vi "Module - RH_BUJAH.vi"() -> ()   [LabVIEW 2019]
uses:
  Control/State - eFGV.ctl
panel:
  out "Site Name":string="RH BUJAH (34.58 kWp)"
  out "STP-04-STATUS":bool
  out "STP-04-B-IDC":dbl caption="B.Idc" format="%.0f A"
  out "STP-04-B-VDC":dbl caption="B.Vdc" format="%.0f V"
  out "STP-04-A-IDC":dbl caption="A.Idc" format="%.0f A"
  out "STP-04-A-VDC":dbl caption="A.Vdc" format="%.0f V"
  out "STP-04-PAC":dbl caption="Pac" format="%#_g W"
  out "BANK-04-TEMP":dbl caption="T_bat" format="%#_g °C"
  out "BANK-04-IDC":dbl caption="I_bat" format="%#_g A"
  out "BANK-04-VDC":dbl caption="V_bat" format="%#_g V"
  out "BANK-04-SOC":dbl caption="SOC" format="%#_g %"
  out "BANK-03-TEMP":dbl caption="T_bat" format="%#_g °C"
  out "BANK-03-IDC":dbl caption="I_bat" format="%#_g A"
  out "BANK-03-VDC":dbl caption="V_bat" format="%#_g V"
  out "BANK-03-SOC":dbl caption="SOC" format="%#_g %"
  out "SI-M-02-STATUS":bool
  out "SI-M-02-FREQ":dbl caption="FREQ" format="%.0f Hz"
  out "SI-M-02-L3":dbl caption="L3" format="%.0f V"
  out "SI-M-02-L2":dbl caption="L2" format="%.0f V"
  out "SI-M-02-L1":dbl caption="L1" format="%.0f V"
  out "SI-M-02-PAC":dbl caption="Pac" format="%.0f W"
  out "STP-03-STATUS":bool
  out "STP-03-B-IDC":dbl caption="B.Idc" format="%.0f A"
  out "STP-03-B-VDC":dbl caption="B.Vdc" format="%.0f V"
  out "STP-03-A-IDC":dbl caption="A.Idc" format="%.0f A"
  out "STP-03-A-VDC":dbl caption="A.Vdc" format="%.0f V"
  out "STP-03-PAC":dbl caption="Pac" format="%#_g W"
  out "PM-01-STATUS":bool
  out "SI-M-01-STATUS":bool
  out "STP-02-STATUS":bool
  out "STP-01-STATUS":bool
  out "BANK-02-TEMP":dbl caption="T_bat" format="%#_g °C"
  out "BANK-02-IDC":dbl caption="I_bat" format="%#_g A"
  out "BANK-02-VDC":dbl caption="V_bat" format="%#_g V"
  out "BANK-02-SOC":dbl caption="SOC" format="%#_g %"
  out "STP-02-B-IDC":dbl caption="B.Idc" format="%.0f A"
  out "STP-02-B-VDC":dbl caption="B.Vdc" format="%.0f V"
  out "STP-02-A-IDC":dbl caption="A.Idc" format="%.0f A"
  out "STP-02-A-VDC":dbl caption="A.Vdc" format="%.0f V"
  out "STP-02-PAC":dbl caption="Pac" format="%#_g W"
  out "PM-01-FREQ":dbl caption="Freq" format="%.0f Hz"
  out "PM-01-IAC":dbl caption="Iac" format="%.0f A"
  out "PM-01-VAC":dbl caption="Vac" format="%.0f V"
  out "PM-01-PAC":dbl caption="Pac" format="%.0f W"
  out "SI-M-01-FREQ":dbl caption="FREQ" format="%.0f Hz"
  out "SI-M-01-L3":dbl caption="L3" format="%.0f V"
  out "SI-M-01-L2":dbl caption="L2" format="%.0f V"
  out "SI-M-01-L1":dbl caption="L1" format="%.0f V"
  out "SI-M-01-PAC":dbl caption="Pac" format="%.0f W"
  out "BANK-01-TEMP":dbl caption="T_bat" format="%#_g °C"
  out "BANK-01-IDC":dbl caption="I_bat" format="%#_g A"
  out "BANK-01-VDC":dbl caption="V_bat" format="%#_g V"
  out "BANK-01-SOC":dbl caption="SOC" format="%#_g %"
  out "STP-01-B-IDC":dbl caption="B.Idc" format="%.0f A"
  out "STP-01-B-VDC":dbl caption="B.Vdc" format="%.0f V"
  out "STP-01-A-IDC":dbl caption="A.Idc" format="%.0f A"
  out "STP-01-A-VDC":dbl caption="A.Vdc" format="%.0f V"
  out "STP-01-PAC":dbl caption="Pac" format="%.0f W"
  # "BANK-1"
  # "BANK-2"
  # "STP2"
  # "BANK-1"
  # "BANK-2"
  # "STP1"
  # "SI-M"
  # "SI-M"
  # "STP3"
  # "STP4"
  # "PM-01"
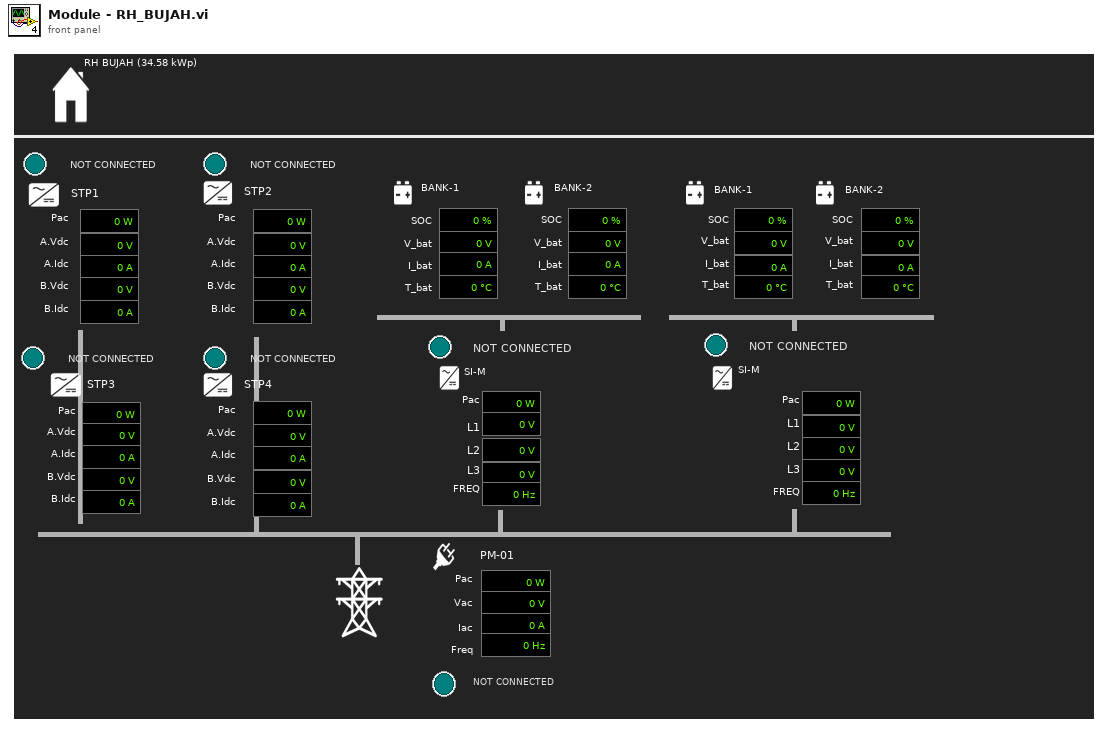
[diagram p1: front panel]
types:
  T1 = typedef "State - eFGV.ctl" = enum16{"Init", "Read", "Write", "Close"}
  T2 = typedef "Device Name.ctl" = enum16{"SB-01", "SB-02", "SB-03", "SB-04", "STP-01", "STP-02", "STP-03", "STP-04", "BANK-01", "BANK-02", "BANK-03", "BANK-04", "SI-M-01", "SI-M-02", "SI-M-03", "SI-M-04", "PM-01", "PM-02", "PM-03", "PM-04"}
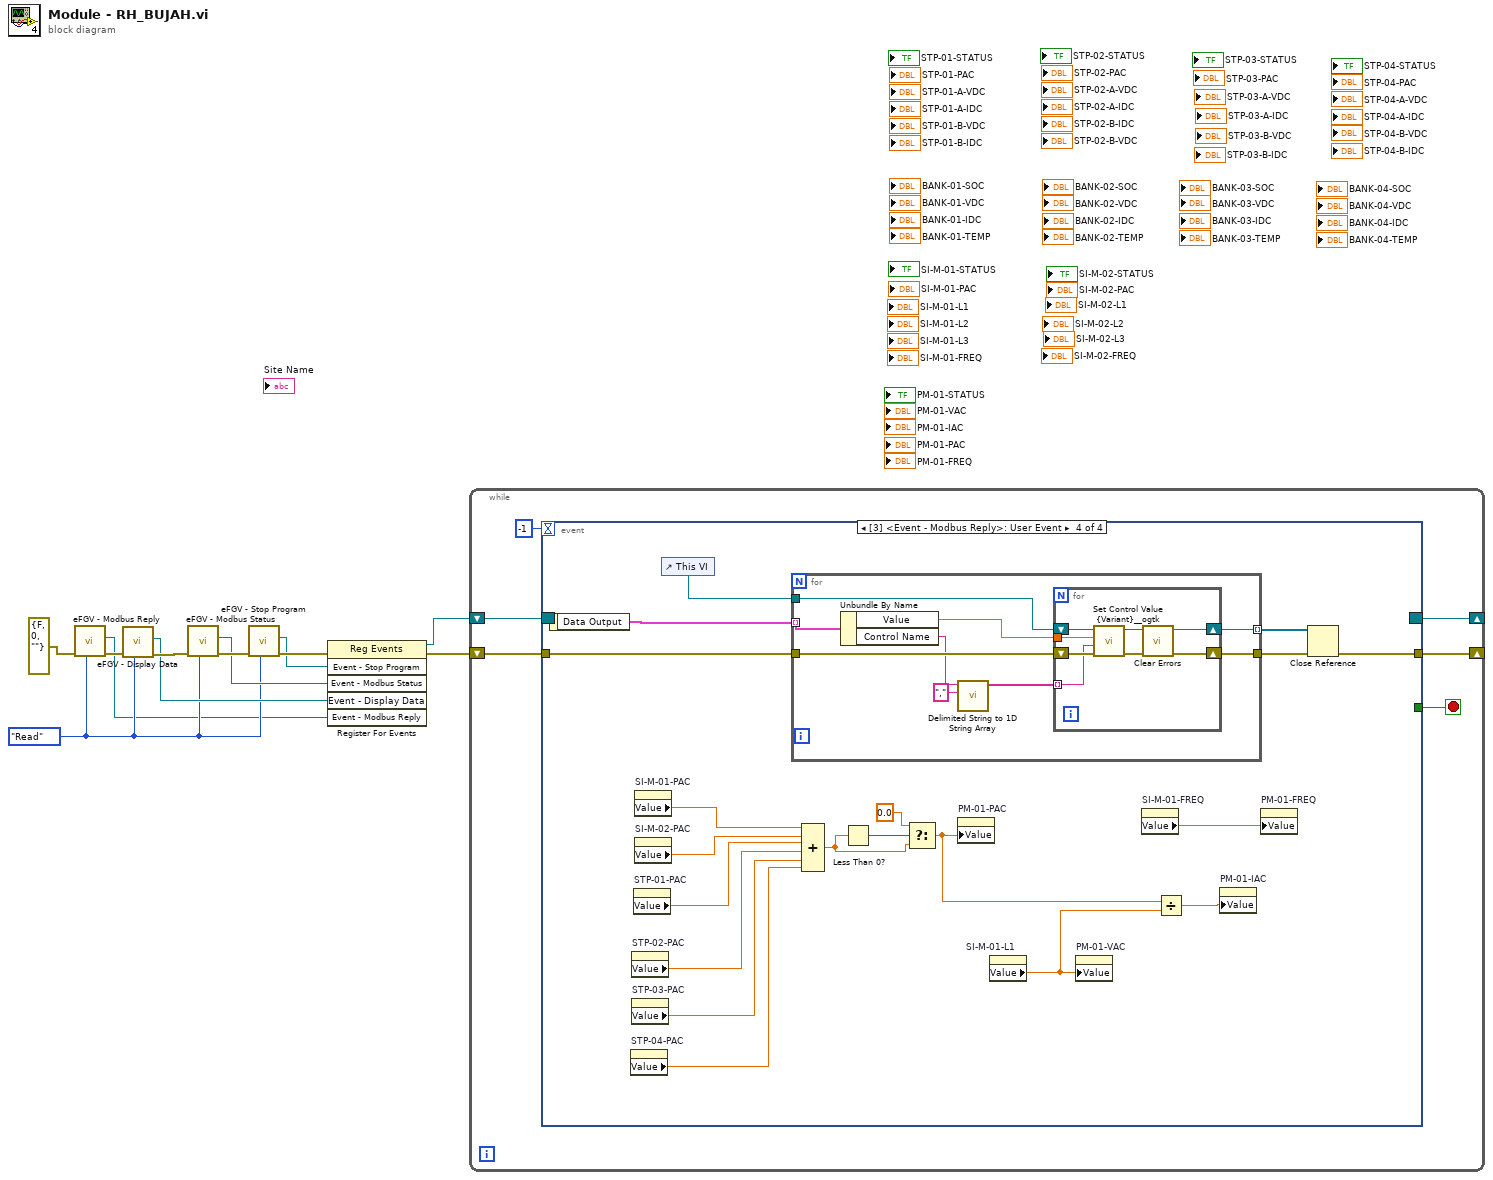
[diagram p0: block diagram]
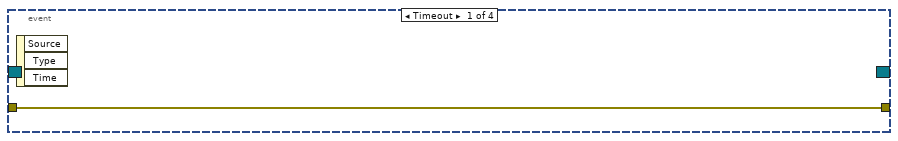
[diagram p2: hidden frame]
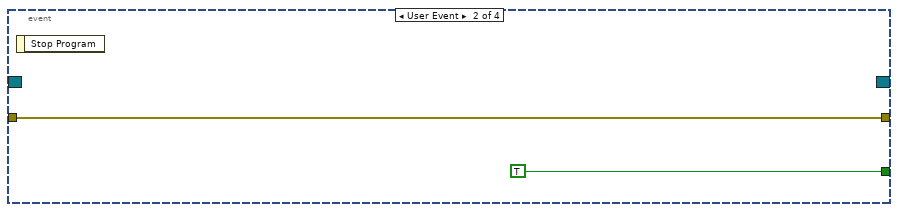
[diagram p3: hidden frame]
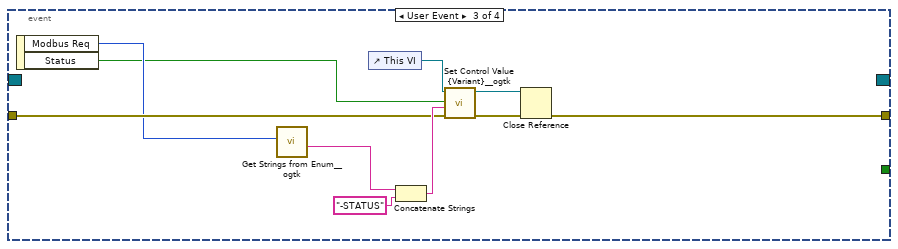
[diagram p4: hidden frame]
diagram:
  w2 = State_-_eFGV."Read" ("State - eFGV")
  n1 = call "eFGV - Modbus Reply.vi"("State - eFGV"=w2, "error in (no error)"=errorcluster {"status"=FALSE, "code"=0, "source"=""}) -> ("error out"=w3:errorcluster, "Event - Modbus Reply"=w1:refnum<user-event>)  [unwired: 8 in]
  n2 = call "eFGV - Display Data.vi"("State - eFGV"=w2, "error in (no error)"=w3) -> ("error out"=w7:errorcluster, "Event - Display Data"=w6:refnum<user-event>)  [unwired: 8 in]
  n3 = call "eFGV - Modbus Status.vi"("State - eFGV"=w2, "error in (no error)"=w7) -> ("error out"=w9:errorcluster, "Event - Modbus Status"=w8:refnum<user-event>)  [unwired: 8 in]
  n4 = call "eFGV - Stop Program.vi"("State - eFGV"=w2, "error in (no error)"=w9) -> ("error out"=w12:errorcluster, "Event - Stop Program"=w11:refnum<user-event>)  [unwired: 8 in]
  n5 = register-events(error in=w12, w11, w8, w6, w1) -> (reference out=w10:refnum<event-registration>, error out=w5:errorcluster)  [unwired: 1 in]
  n6 = while {
    shift-right: [w17] -> _
    shift-left: w10 -> [w18]
    shift-right: [w14] -> _
    shift-left: w5 -> [w13]
    stop <- w16 stop-if-true
    n7 = event shown="[3] <Event - Modbus Reply>: User Event" {
      selector: w18 -> [_ _ _ _]
      dyn-events: [_ _ _ _] -> w17
      timeout: -1 -> [_ _ _ _]
      tunnel: w13 -> [w19 w20 w25 w45]
      tunnel: [_ TRUE _ _] -> w16
      tunnel: [w19 w20 w22 w47] -> w14
      event Timeout {
        n8 = event-data() -> ()  [unwired: 1 in, 3 out]
      }
      event User Event {
        n9 = event-data() -> ()  [unwired: 1 in, 1 out]
      }
      event User Event {
        n10 = event-data() -> ("Modbus Req"=w24:T2, "Status"=w23:bool)  [unwired: 1 in]
        n11 = call "Get Strings from Enum__ogtk.vi"("Enum"=w24) -> ("String Value"=w27:string)  [unwired: 7 in, 3 out]
        n12 = control-ref of="This VI"() -> (w31:refnum<vi>)
        n13 = Concatenate Strings(w27, "-STATUS" ("string")) -> (w30:string)
        n14 = call "Set Control Value {Variant}__ogtk.vi"("error in (no error)"=w25, "Control Name (\"\": use variant name)"=w30, "Value"=w23, "VI Refnum"=w31) -> ("error out"=w29:errorcluster, "VI Refnum dup"=w28:refnum<vi>)  [unwired: 6 in]
        n15 = Close Reference(reference=w28, error in (no error)=w29) -> (error out=w22:errorcluster)
      }
      event User Event {
        n16 = event-data() -> ("Data Output"=w46:cluster{"Control Name":string, "Value":dbl}[])  [unwired: 1 in]
        n17 = property on="STP-04-PAC" class="DigNum (strict)"() -> ("Value"=w32:dbl)  [unwired: 2 in, 2 out]
        n18 = property on="STP-02-PAC" class="DigNum (strict)"() -> ("Value"=w34:dbl)  [unwired: 2 in, 2 out]
        n19 = property on="STP-03-PAC" class="DigNum (strict)"() -> ("Value"=w33:dbl)  [unwired: 2 in, 2 out]
        n20 = property on="STP-01-PAC" class="DigNum (strict)"() -> ("Value"=w41:dbl)  [unwired: 2 in, 2 out]
        n21 = property on="SI-M-01-PAC" class="DigNum (strict)"() -> ("Value"=w43:dbl)  [unwired: 2 in, 2 out]
        n22 = property on="SI-M-02-PAC" class="DigNum (strict)"() -> ("Value"=w42:dbl)  [unwired: 2 in, 2 out]
        n23 = control-ref of="This VI"() -> (w50:refnum<vi>)
        n24 = for {
          tunnel: w50 -> [w59]
          tunnel: w45 -> [w58]
          tunnel: [w57] -> w49
          tunnel: [w56] -> w48 mode=indexing
          tunnel: w46 -> [w55] mode=indexing
          n25 = Unbundle By Name(w55) -> ("Value"=w54:dbl, "Control Name"=w53:string)
          n26 = call <vilib>:"Delimited String to 1D String Array.vi"("delimiter"=",", "delimited string"=w53) -> ("string array"=w51:string[])  [unwired: 9 in]
          n27 = for {
            tunnel: w54 -> [w62]
            shift-right: [w63] -> w56
            shift-left: w59 -> [w66]
            shift-right: [w60] -> w57
            shift-left: w58 -> [w65]
            tunnel: w51 -> [w61] mode=indexing
            n28 = call "Set Control Value {Variant}__ogtk.vi"("error in (no error)"=w65, "Control Name (\"\": use variant name)"=w61, "Value"=w62, "VI Refnum"=w66) -> ("error out"=w64:errorcluster, "VI Refnum dup"=w63:refnum<vi>)  [unwired: 6 in]
            n29 = call <vilib>:"Clear Errors.vi"("error in (no error)"=w64) -> ("error out"=w60:errorcluster)  [unwired: 5 in, 1 out]
          }
        }
        n30 = Compound Arithmetic op=ADD(w43, w42, w41, w34, w33, w32) -> (w39:dbl)
        n31 = Less Than 0?(x=w39) -> (x < 0?=w40:bool)
        n32 = Select(t=0.0, s=w40, f=w39) -> (s? t:f=w36:dbl)
        n33 = property on="PM-01-PAC" class="DigNum (strict)"("Value"=w36) -> ()  [unwired: 2 in, 2 out]
        n34 = property on="SI-M-01-L1" class="DigNum (strict)"() -> ("Value"=w35:dbl)  [unwired: 2 in, 2 out]
        n35 = property on="PM-01-VAC" class="DigNum (strict)"("Value"=w35) -> ()  [unwired: 2 in, 2 out]
        n36 = property on="SI-M-01-FREQ" class="DigNum (strict)"() -> ("Value"=w44:dbl)  [unwired: 2 in, 2 out]
        n37 = Divide(x=w36, y=w35) -> (x/y=w37:dbl)
        n38 = property on="PM-01-IAC" class="DigNum (strict)"("Value"=w37) -> ()  [unwired: 2 in, 2 out]
        n39 = property on="PM-01-FREQ" class="DigNum (strict)"("Value"=w44) -> ()  [unwired: 2 in, 2 out]
        n40 = Close Reference(reference=w48, error in (no error)=w49) -> (error out=w47:errorcluster)
      }
    }
  }
